vi "MSE PtByPt.vi"(2 "initialize":bool, 3 "sample length":i32=100, 4 "y":dbl format="%0.2f", 5 "x":dbl format="%0.2f") -> (0 "error":i32, 1 "mse":dbl format="%0.2f")   [LabVIEW 2020, in "NI_PtbyPt.lvlib"]
doc: "Computes the mean square error (<B>mse</B>) of <B>x</B> and <B>y</B>."
uses:
  NI_PtbyPt.lvlib
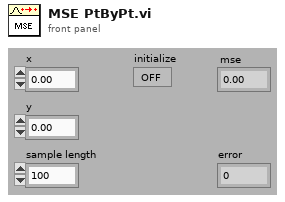
[diagram p1: front panel]
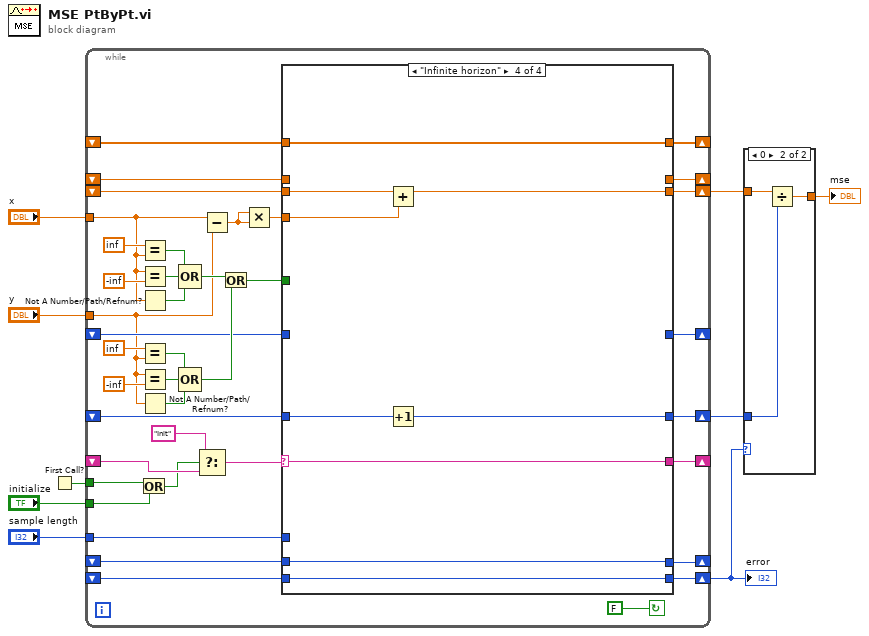
[diagram p0: block diagram]
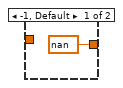
[diagram p2: hidden frame]
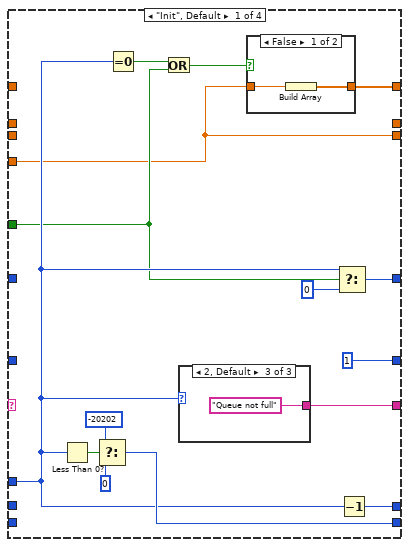
[diagram p3: hidden frame]
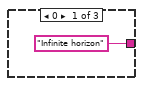
[diagram p5: hidden frame]
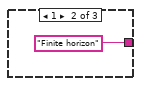
[diagram p6: hidden frame]
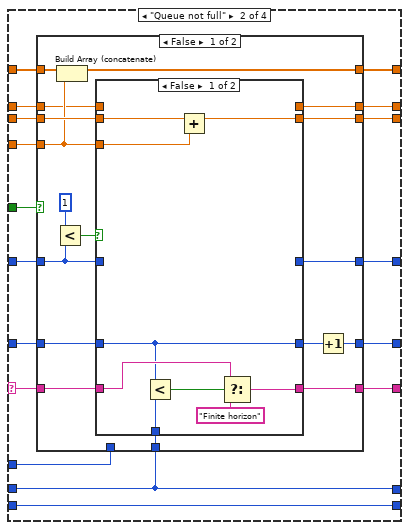
[diagram p7: hidden frame]
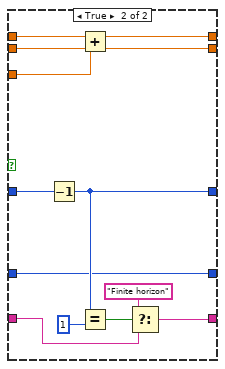
[diagram p8: hidden frame]
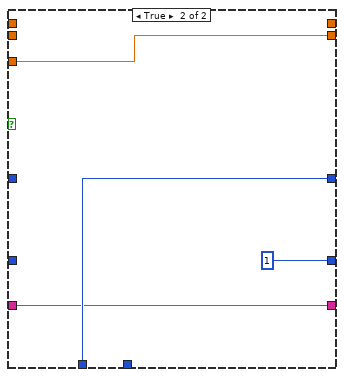
[diagram p9: hidden frame]
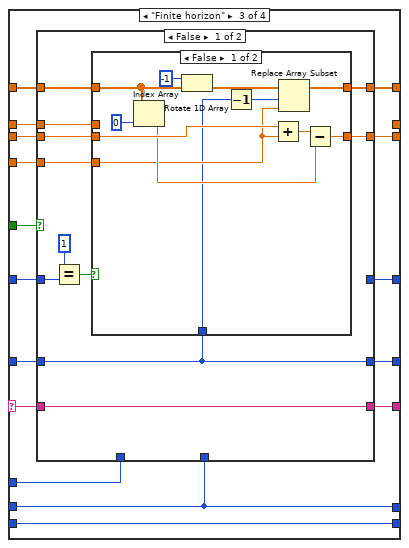
[diagram p10: hidden frame]
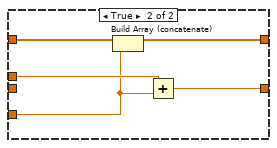
[diagram p11: hidden frame]
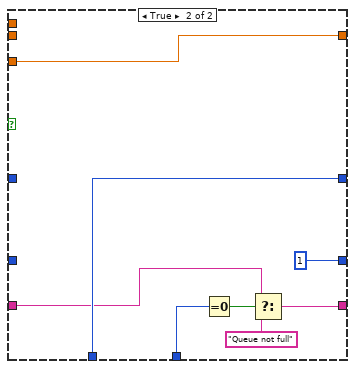
[diagram p12: hidden frame]
diagram:
  n1 = First Call?() -> (First Call?: T/F=w7:bool)
  n2 = while {
    tunnel: w7 -> [w36]
    shift-left: _ -> [w38]
    shift-right: [w39] -> _
    shift-left: _ -> [w40]
    shift-right: [w41] -> w6
    shift-left: _ -> [w43]
    shift-right: [w42] -> _
    shift-left: _ -> [w45]
    shift-right: [w46] -> w8
    shift-left: _ -> [w49]
    shift-right: [w44] -> _
    shift-right: [w19] -> _
    shift-left: _ -> [w18]
    shift-right: [w17] -> _
    shift-left: _ -> [w16]
    shift-right: [w15] -> w5
    shift-left: _ -> [w14]
    tunnel: "x" -> [w13]
    tunnel: "y" -> [w12]
    tunnel: "sample length" -> [w11]
    tunnel: "initialize" -> [w10]
    stop <- FALSE continue-if-true
    n3 = Or(x=w36, y=w10) -> (x .or. y?=w35:bool)
    n4 = Equal?(x=inf, y=w13) -> (x = y?=w29:bool)
    n5 = Equal?(x=w13, y=-inf) -> (x = y?=w30:bool)
    n6 = Not A Number/Path/Refnum?(number/path/refnum=w13) -> (NaN/Path/Refnum?=w28:bool)
    n7 = Equal?(x=inf, y=w12) -> (x = y?=w26:bool)
    n8 = Equal?(x=w12, y=-inf) -> (x = y?=w25:bool)
    n9 = Not A Number/Path/Refnum?(number/path/refnum=w12) -> (NaN/Path/Refnum?=w27:bool)
    n10 = Compound Arithmetic op=OR(w29, w30, w28) -> (w22:bool)
    n11 = Compound Arithmetic op=OR(w26, w25, w27) -> (w21:bool)
    n12 = Select(t="Init", s=w35, f=w49) -> (s? t:f=w47:string)
    n13 = Subtract(x=w13, y=w12) -> (x-y=w34:dbl)
    n14 = Or(x=w22, y=w21) -> (x .or. y?=w20:bool)
    n15 = Multiply(x=w34, y=w34) -> (x*y=w33:dbl)
    n16 = case shown="\"Infinite horizon\"" w47 {
      selector: w47 -> [_ w83 w139 w188]
      tunnel: [1 w77 w136 w181] -> w46
      tunnel: w45 -> [_ w84 w137 w189]
      tunnel: [w56 w82 w138 w188] -> w44
      tunnel: w43 -> [_ w86 w143 w183]
      tunnel: [w51 w85 w144 w183] -> w42
      tunnel: w11 -> [w55 w71 w132 _]
      tunnel: [w50 w81 w141 w186] -> w41
      tunnel: w40 -> [_ w80 w142 w187]
      tunnel: [w60 w79 w130 w185] -> w39
      tunnel: w38 -> [_ w79 w130 w185]
      tunnel: w33 -> [w50 w78 w140 w184]
      tunnel: w20 -> [w53 w76 w135 _]
      tunnel: [w59 w72 w131 _] -> w19
      tunnel: w18 -> [_ w73 w134 _]
      tunnel: [_ w75 _ _] -> w17
      tunnel: w16 -> [_ w74 w133 _]
      tunnel: [w57 w70 w129 w182] -> w15
      tunnel: w14 -> [_ w70 w129 w182]
      frame "Init", Default {
        n17 = Less Than 0?(x=w55) -> (x < 0?=w61:bool)
        n18 = Select(t=-20202, s=w61, f=0) -> (s? t:f=w57:i32)
        n19 = Equal To 0?(x=w55) -> (x = 0?=w54:bool)
        n20 = Or(x=w54, y=w53) -> (x .or. y?=w52:bool)
        n21 = case shown="2, Default" w55 {
          tunnel: ["Infinite horizon" "Finite horizon" "Queue not full" ("f")] -> w56
          frame 0 {
          }
          frame 1 {
          }
          frame 2, Default {
          }
        }
        n22 = case shown="False" w52 {
          tunnel: [w66 _] -> w51
          tunnel: w50 -> [w65 _]
          frame False {
            n23 = Build Array(w65) -> (w66:dbl[])
          }
          frame True {
          }
        }
        n24 = Select(t=w55, s=w53, f=0) -> (s? t:f=w59:i32)
        n25 = Decrement(x=w55) -> (x-1=w60:i32)
      }
      frame "Queue not full" {
        n26 = case shown="False" w76 {
          tunnel: w86 -> [w103 _]
          tunnel: [w102 _] -> w85
          tunnel: w84 -> [w101 _]
          tunnel: w83 -> [w100 w127]
          tunnel: [w99 w127] -> w82
          tunnel: [w98 w125] -> w81
          tunnel: w80 -> [w97 _]
          tunnel: w79 -> [w96 _]
          tunnel: w78 -> [w95 w125]
          tunnel: [w94 1] -> w77
          tunnel: [w92 _] -> w75
          tunnel: w74 -> [w91 _]
          tunnel: w73 -> [w88 _]
          tunnel: [w90 w128] -> w72
          tunnel: w71 -> [_ w128]
          frame False {
            n27 = Less?(x=1, y=w88) -> (x < y?=w87:bool)
            n28 = Build Array (concatenate)(w103, w95) -> (w102:dbl[])
            n29 = case shown="False" w87 {
              tunnel: w101 -> [w104 w115]
              tunnel: w100 -> [w111 w113]
              tunnel: [w109 w114] -> w99
              tunnel: [w108 w121] -> w98
              tunnel: w97 -> [w107 w121]
              tunnel: w96 -> [w106 _]
              tunnel: w95 -> [w105 w124]
              tunnel: [w104 w115] -> w93
              tunnel: [_ w123] -> w92
              tunnel: w91 -> [_ w122]
              tunnel: w88 -> [_ w117]
              tunnel: [_ w116] -> w90
              frame False {
                n30 = Less?(x=w104, y=w106) -> (x < y?=w112:bool)
                n31 = Add(x=w107, y=w105) -> (x+y=w108:dbl)
                n32 = Select(t=w111, s=w112, f="Finite horizon") -> (s? t:f=w109:string)
              }
              frame True {
                n33 = Decrement(x=w117) -> (x-1=w116:i32)
                n34 = Add(x=w122, y=w124) -> (x+y=w123:dbl)
                n35 = Equal?(x=w116, y=1) -> (x = y?=w120:bool)
                n36 = Select(t="Finite horizon" ("f"), s=w120, f=w113) -> (s? t:f=w114:string)
              }
            }
            n37 = Increment(x=w93) -> (x+1=w94:i32)
          }
          frame True {
          }
        }
      }
      frame "Finite horizon" {
        n38 = case shown="False" w135 {
          tunnel: [w155 _] -> w144
          tunnel: w143 -> [w154 _]
          tunnel: w142 -> [w153 _]
          tunnel: [w152 w180] -> w141
          tunnel: w137 -> [w149 _]
          tunnel: w140 -> [w151 w180]
          tunnel: w139 -> [w150 w174]
          tunnel: [w150 w175] -> w138
          tunnel: [w149 1] -> w136
          tunnel: w134 -> [w147 _]
          tunnel: w133 -> [w145 _]
          tunnel: w132 -> [_ w179]
          tunnel: [_ w179] -> w131
          tunnel: w130 -> [_ w173]
          frame False {
            n39 = Equal?(x=1, y=w147) -> (x = y?=w146:bool)
            n40 = case shown="False" w146 {
              tunnel: [w163 w171] -> w155
              tunnel: w154 -> [w162 w172]
              tunnel: w153 -> [w161 _]
              tunnel: [w159 w170] -> w152
              tunnel: w151 -> [w157 w168]
              tunnel: w149 -> [w156 _]
              tunnel: w145 -> [_ w169]
              frame False {
                n41 = Index Array(array=w162, index=0 ("Index")) -> (element=w158:dbl)
                n42 = Rotate 1D Array(1:w162, 2:i16 -1 ("n")) -> (0:w165:dbl[])
                n43 = Decrement(x=w156) -> (x-1=w164:i32)
                n44 = Add(x=w161, y=w157) -> (x+y=w160:dbl)
                n45 = Replace Array Subset(array=w165, new element=w157, index=w164) -> (w163:dbl[])
                n46 = Subtract(x=w160, y=w158) -> (x-y=w159:dbl)
              }
              frame True {
                n47 = Build Array (concatenate)(w172, w168) -> (w171:dbl[])
                n48 = Add(x=w169, y=w168) -> (x+y=w170:dbl)
              }
            }
          }
          frame True {
            n49 = Equal To 0?(x=w173) -> (x = 0?=w178:bool)
            n50 = Select(t=w174, s=w178, f="Queue not full") -> (s? t:f=w175:string)
          }
        }
      }
      frame "Infinite horizon" {
        n51 = Add(x=w187, y=w184) -> (x+y=w186:dbl)
        n52 = Increment(x=w189) -> (x+1=w181:i32)
      }
    }
  }
  "error" <- w5
  n53 = case shown="0" w5 {
    tunnel: [nan w193] -> w9
    tunnel: w8 -> [_ w192]
    tunnel: w6 -> [_ w191]
    frame -1, Default {
    }
    frame 0 {
      n54 = Divide(x=w191, y=w192) -> (x/y=w193:dbl)
    }
  }
  "mse" <- w9
